vi "Get PlotConfig.vi"(8 "error in (no error)":errorcluster, 9 "request timeout in ms (-1)":i32=-1, 11 "BluePlotHandle in":refnum<class "BluePlotHandle.lvclass">) -> (0 "error out":errorcluster, 2 "Plot config":T1={"plots"=[], "X-axis"={"Name Label.Text"="", "Style"=0, "Tick Colors:Minor Tick Color"=0, "Tick Colors:Tick Color"=0, "Marker Colors:Text Color"=0, "Grid Colors:Major Color"=0, "Grid Colors:Minor Color"=0, "Mapping Mode"=0, "Flipped"=FALSE, "Name Label.Visible"=FALSE, "Name Label.Text Colors:Text Color"=0, "Scale Fit"=0, "Editable"=FALSE, "Range:Maximum"=0.0, "Range:Minimum"=0.0, "Offset and Multiplier:Multiplier"=0.0, "Offset and Multiplier:Offset"=0.0, "Name Label.Font:Size"=0, "Marker.Font:Size"=0, "Uniform Marker Spacing?"=TRUE, "Format String"=""}, "Y-axes"=[], "General"={"Title"="", "Time to Plot"=1800.0, "Title.Visible"=FALSE, "Sidebar.Visible"=FALSE, "Plot Area:Colors:BG Color"=0}} {"General"."Time to Plot" format="%<%M:%S>t"}, 3 "BluePlotHandle out":refnum<class "BluePlotHandle.lvclass">)   [LabVIEW 2021, in "BluePlot.lvlib" / "BluePlotHandle.lvclass"]
doc: "This will fetch a large cluster which represents the \"plot config\".\n\nThe intent here is to enable users to easily save/load plot configurations.\nThe plot configuration captures all plot settings/properties which can be modified by a user at the user interface.\nThis is a large cluster because, frankly, there are alot of user-adjustable properties. Which is kinda what makes this package valuable.\n\nI recommend just JDP JSONtext to serialize this cluster to/from JSON in order to save this as a configuration file on disk."
uses:
  BluePlotHandle.lvclass
  TypeDefs/plot load data V2.ctl
  TypeDefs/plot properties V2.ctl
  TypeDefs/plot attributes V2.ctl
  TypeDefs/Plot scale axis properties.ctl
  TypeDefs/Plot general properties.ctl
  BluePlotHandle.lvclass/BluePlotHandle.ctl
  TypeDefs/plot handle queue data.ctl
  TypeDefs/Plot QSM action.ctl
  BluePlot.lvlib
  <vilib>/Futures/Futures/Futures.lvlib
  <vilib>/Futures/Futures/Future/Future.lvclass
  <vilib>/Futures/Futures/Promise/Promise.lvclass
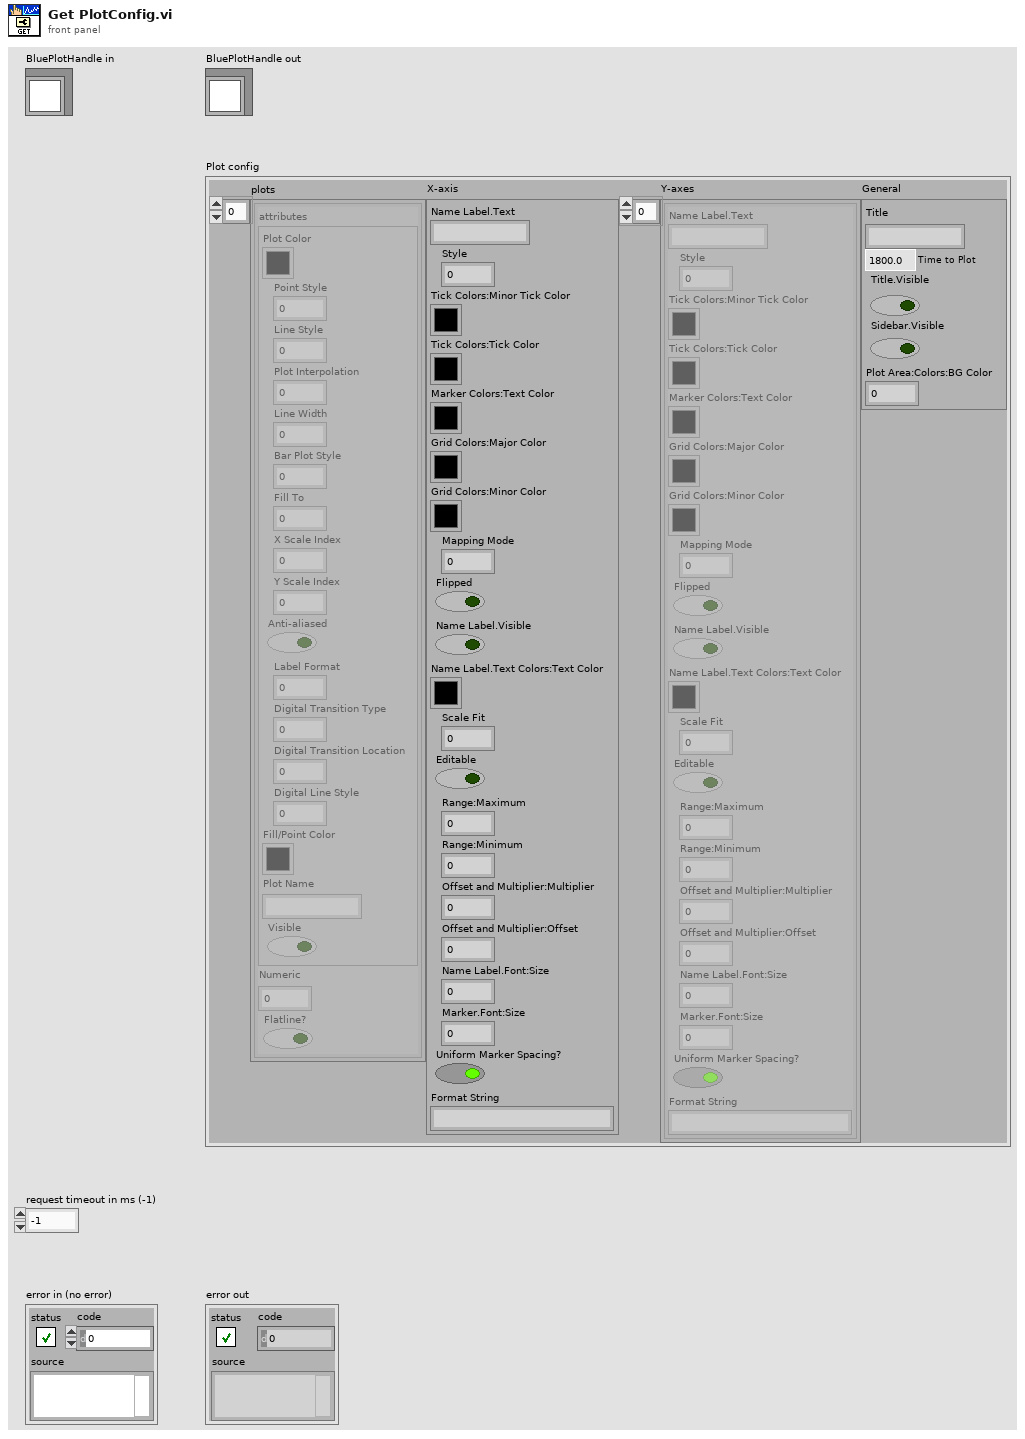
[diagram p1: front panel]
types:
  T1 = typedef "BluePlot.lvlib/plot load data V2.ctl" = cluster{"plots":T2[], "X-axis":T4, "Y-axes":T4[], "General":T5}
  T2 = typedef "BluePlot.lvlib/plot properties V2.ctl" = cluster{"attributes":T3, "Numeric":dbl, "Flatline?":bool}
  T3 = typedef "BluePlot.lvlib/plot attributes V2.ctl" = cluster{"Plot Color":u32, "Point Style":u8, "Line Style":u8, "Plot Interpolation":u8, "Line Width":u8, "Bar Plot Style":u8, "Fill To":i16, "X Scale Index":u32, "Y Scale Index":u32, "Anti-aliased":bool, "Label Format":u8, "Digital Transition Type":u8, "Digital Transition Location":u8, "Digital Line Style":u8, "Fill/Point Color":u32, "Plot Name":string, "Visible":bool}
  T4 = typedef "BluePlot.lvlib/Plot scale axis properties.ctl" = cluster{"Name Label.Text":string, "Style":u8, "Tick Colors:Minor Tick Color":u32, "Tick Colors:Tick Color":u32, "Marker Colors:Text Color":u32, "Grid Colors:Major Color":u32, "Grid Colors:Minor Color":u32, "Mapping Mode":u8, "Flipped":bool, "Name Label.Visible":bool, "Name Label.Text Colors:Text Color":u32, "Scale Fit":u8, "Editable":bool, "Range:Maximum":dbl, "Range:Minimum":dbl, "Offset and Multiplier:Multiplier":dbl, "Offset and Multiplier:Offset":dbl, "Name Label.Font:Size":u32, "Marker.Font:Size":u32, "Uniform Marker Spacing?":bool, "Format String":string}
  T5 = typedef "BluePlot.lvlib/Plot general properties.ctl" = cluster{"Title":string, "Time to Plot":dbl, "Title.Visible":bool, "Sidebar.Visible":bool, "Plot Area:Colors:BG Color":u32}
  T6 = typedef "BluePlot.lvlib/Plot QSM action.ctl" = enum16{"start updating", "stop updating", "Shutdown", "Update", "Init", "Get Config", "Load Config"}
  T7 = typedef "BluePlot.lvlib/plot handle queue data.ctl" = cluster{"action":T6, "data":variant}
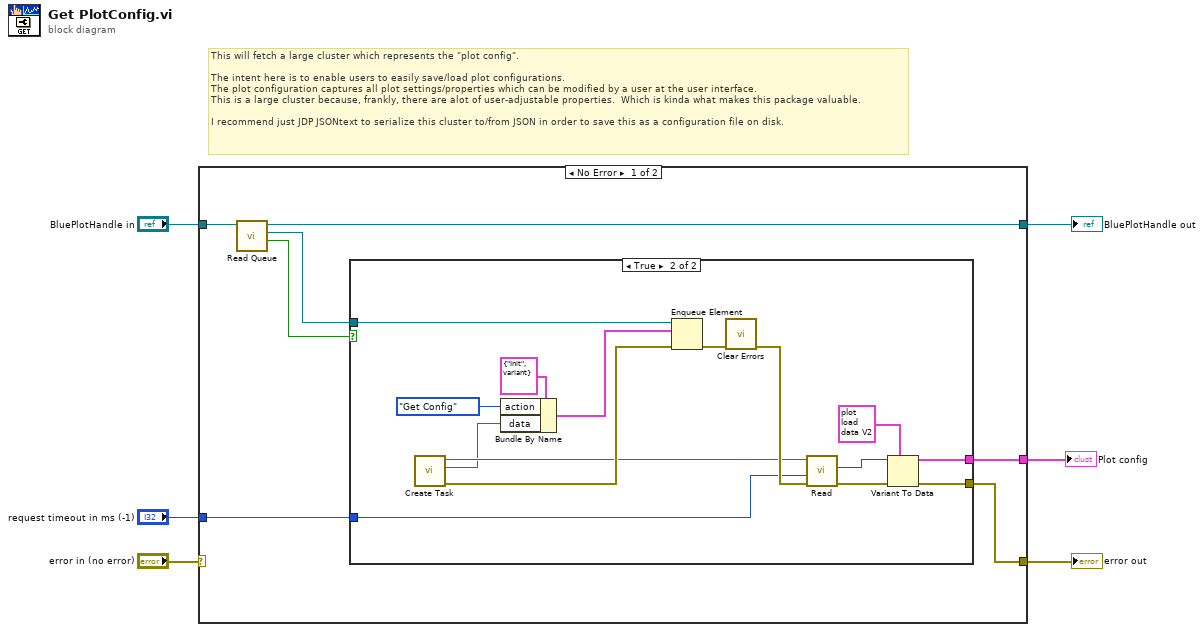
[diagram p0: block diagram]
diagram:
  # "This will fetch a large cluster which represents the \"plot config\".\n\nThe intent here is to enable users to easily save/load plot configurations.\nThe plot configuration captures all plot settings/properties which can be modified by a user at the user interface.\nThis is a large cluster because, frankly, there are alot of user-adjustable properties.  Which is kinda what makes this package valuable.\n\nI recommend just JDP JSONtext to serialize this cluster to/from JSON in order to save this as a configuration file on disk."
  n1 = case shown="No Error" "error in (no error)" {
    selector: "error in (no error)" -> [_ w30]
    tunnel: "BluePlotHandle in" -> [w12 w29]
    tunnel: "request timeout in ms (-1)" -> [w10 _]
    tunnel: [w9 w30] -> w4
    tunnel: [w8 w29] -> w2
    tunnel: [w7 _] -> w1
    frame No Error {
      n2 = call "Read Queue.vi"("BluePlotHandle in"=w12) -> ("Valid?"=w13:bool, "Queue"=w11:refnum<queue>, "BluePlotHandle out"=w8:refnum<class "BluePlotHandle.lvclass">)  [unwired: 8 in]
      n3 = case shown="True" w13 {
        tunnel: w11 -> [_ w28]
        tunnel: w10 -> [_ w19]
        tunnel: [_ w15] -> w9
        tunnel: [_ w14] -> w7
        frame False {
        }
        frame True {
          n4 = call <vilib>:"Create Task.vi"() -> ("error out"=w23:errorcluster, "Promise out"=w20:refnum<class "Promise.lvclass">, "Future out"=w21:refnum<class "Future.lvclass">)  [unwired: 9 in]
          n5 = Bundle By Name(cluster=T7 {"action"=enum."Init", "data"=variant} ("element"), "action"=Plot_QSM_action."Get Config", "data"=w20) -> (w25:T7)
          n6 = Enqueue Element(queue=w28, element=w25, error in (no error)=w23) -> (error out=w24:errorcluster)  [unwired: 1 in, 2 out]
          n7 = call <vilib>:"Clear Errors.vi"("error in (no error)"=w24) -> ("error out"=w22:errorcluster)  [unwired: 5 in, 1 out]
          n8 = call <vilib>:"Read.vi"("error in (no error)"=w22, "timeout in ms (60 sec)"=w19, "Future in"=w21) -> ("error out"=w18:errorcluster, "Result value"=w16:variant)  [unwired: 5 in, 2 out]
          n9 = Variant To Data(error in=w18, type=T1 {"plots"=[], "X-axis"={"Name Label.Text"="", "Style"=0, "Tick Colors:Minor Tick Color"=0, "Tick Colors:Tick Color"=0, "Marker Colors:Text Color"=0, "Grid Colors:Major Color"=0, "Grid Colors:Minor Color"=0, "Mapping Mode"=0, "Flipped"=FALSE, "Name Label.Visible"=FALSE, "Name Label.Text Colors:Text Color"=0, "Scale Fit"=0, "Editable"=FALSE, "Range:Maximum"=0.0, "Range:Minimum"=0.0, "Offset and Multiplier:Multiplier"=0.0, "Offset and Multiplier:Offset"=0.0, "Name Label.Font:Size"=0, "Marker.Font:Size"=0, "Uniform Marker Spacing?"=TRUE, "Format String"=""}, "Y-axes"=[], "General"={"Title"="", "Time to Plot"=1800.0, "Title.Visible"=FALSE, "Sidebar.Visible"=FALSE, "Plot Area:Colors:BG Color"=0}} ("Plot config"), Variant=w16) -> (data=w14:T1, error out=w15:errorcluster)
        }
      }
    }
    frame Error {
    }
  }
  "BluePlotHandle out" <- w2
  "error out" <- w4
  "Plot config" <- w1
